vi "Network Engine.vi"(8 "error in (no error)":errorcluster, 11 "Variables":T1) -> (0 "error out":errorcluster)   [LabVIEW 2019, in "Protection and Counter Addon Engine.lvlib"]
uses:
  Protection and Counter Addon Engine.lvlib
  Types/RT Async Engine Variables.ctl
  <vilib>/NI/NIVS Inline Async API/_VS Inline Async API/Process/Process.lvclass
  <vilib>/NI/NI VeriStand Addon Network Comm/Engine/VeriStand Comm.lvclass
  Types/RT Data References.ctl
  <vilib>/NI/NIVS Inline Async API/_Data Access Engine/Data Access Engine/Types/Write.DVR.ctl
  <vilib>/NI/NIVS Inline Async API/_Data Access Engine/Access Type Classes/Write/Write.lvclass
  <vilib>/NI/NIVS Inline Async API/_Data Access Engine/Data Access Engine/Types/Read.DVR.ctl
  <vilib>/NI/NIVS Inline Async API/_Data Access Engine/Access Type Classes/Read/Read.lvclass
  Types/RT Async Engine Settings.ctl
  SubModules/Frame Protection Support/Source/Engine/Types/RT Frame Settings.ctl
  SubModules/Frame Protection Support/Source/Shared/Types/Exported Frame Type.ctl
  SubModules/Frame Protection Support/Source/Engine/Types/RT Protection Configuration.ctl
  SubModules/Frame Protection Support/Source/Shared/Types/Protection Type.ctl
  SubModules/Frame Protection Support/Source/Shared/Types/XNET Signal Configuration.ctl
  SubModules/Frame Protection Support/Source/Shared/Types/Exported Counter Settings.ctl
  SubModules/Frame Protection Support/Source/Shared/Types/Exported Event Trigger Type.ctl
  <vilib>/NI/NI VeriStand Addon Network Comm/Engine/VeriStand Comm.lvclass/VeriStand Comm.ctl
  <vilib>/NI/NIVS Inline Async API/_VS Inline Async API/Process/Process.lvclass/Process.ctl
  <vilib>/xnet/xnet.llb/XNET Frame CAN.ctl
  <vilib>/xnet/xnet.llb/XNET Frame Type CAN.ctl
  <vilib>/NI/NI VeriStand Addon Network Comm/Engine/_SubVIs/Comm Connection Engine.vi
  <vilib>/NI/NI VeriStand Addon Network Comm/Engine/_SubVIs/Comm Command Engine.vi
  <vilib>/NI/NIVS Inline Async API/_VS Inline Async API/Error Handling Process/SubVIs/Error.ConvertArray.vi
  <vilib>/NI/AMC/Read Next Message.vi
  <vilib>/NI/Tools/Keyed Array/Index.vi
  <vilib>/NI/AMC/Send Local Message.vi
  <vilib>/NI/STM/Connection Manager/TCP/Advanced/TCP Connection Manager (By Reference).vi
  <vilib>/Utility/error.llb/Clear Errors.vi
  <vilib>/NI/STM/Get Connection Reference.vi
  <vilib>/NI/STM/TCP/Get Connection Reference (TCP).vi
  <vilib>/NI/STM/Read Meta Data.vi
  <vilib>/NI/STM/TCP/Read Meta Data (TCP Ref).vi
  <vilib>/NI/Tools/Keyed Array/Add.vi
  <vilib>/NI/STM/Connection Manager/TCP/Advanced/TCP Check Connection (By Reference).vi
  <vilib>/NI/AMC/Read Termination Message.vi
  <vilib>/NI/Tools/Keyed Array/Map String.vi
  <vilib>/NI/AMC/Create Single Message.vi
  <vilib>/NI/AMC/Update Message Routing Info.vi
  <vilib>/NI/STM/SubVIs/Generate STM Error.vi
  <vilib>/NI/Tools/String/Get Case Matching.vi
  <vilib>/NI/STM/Read Message.vi
  <vilib>/NI/STM/TCP/Read Message (TCP).vi
  <vilib>/NI/AMC/Send Message.vi
  <vilib>/NI/NI VeriStand Addon Network Comm/Shared/Comm Constants.vi
  <vilib>/NI/AMC/Create Message Queue.vi
  <vilib>/NI/AMC/Globals.vi
  <vilib>/NI/STM/Write Message.vi
  <vilib>/NI/STM/TCP/Write Message (TCP).vi
  <vilib>/NI/AMC/Destroy Message Queue.vi
  <vilib>/Utility/SystemLogging/Write to System Log.vi
  <vilib>/NI/STM/TCP/Read Meta Data (TCP Clst).vi
  <vilib>/xnet/xnet.llb/XNET Write (Frame CAN).vi
  SubModules/Frame Protection Support/Source/Shared/Protection and Counter Support Shared.lvlib
  SubModules/Frame Protection Support/Source/Engine/Protection and Counter Support Engine.lvlib
  <vilib>/NI/NIVS Inline Async API/_Data Access Engine/Data Access Engine/Data Access Engine.lvclass
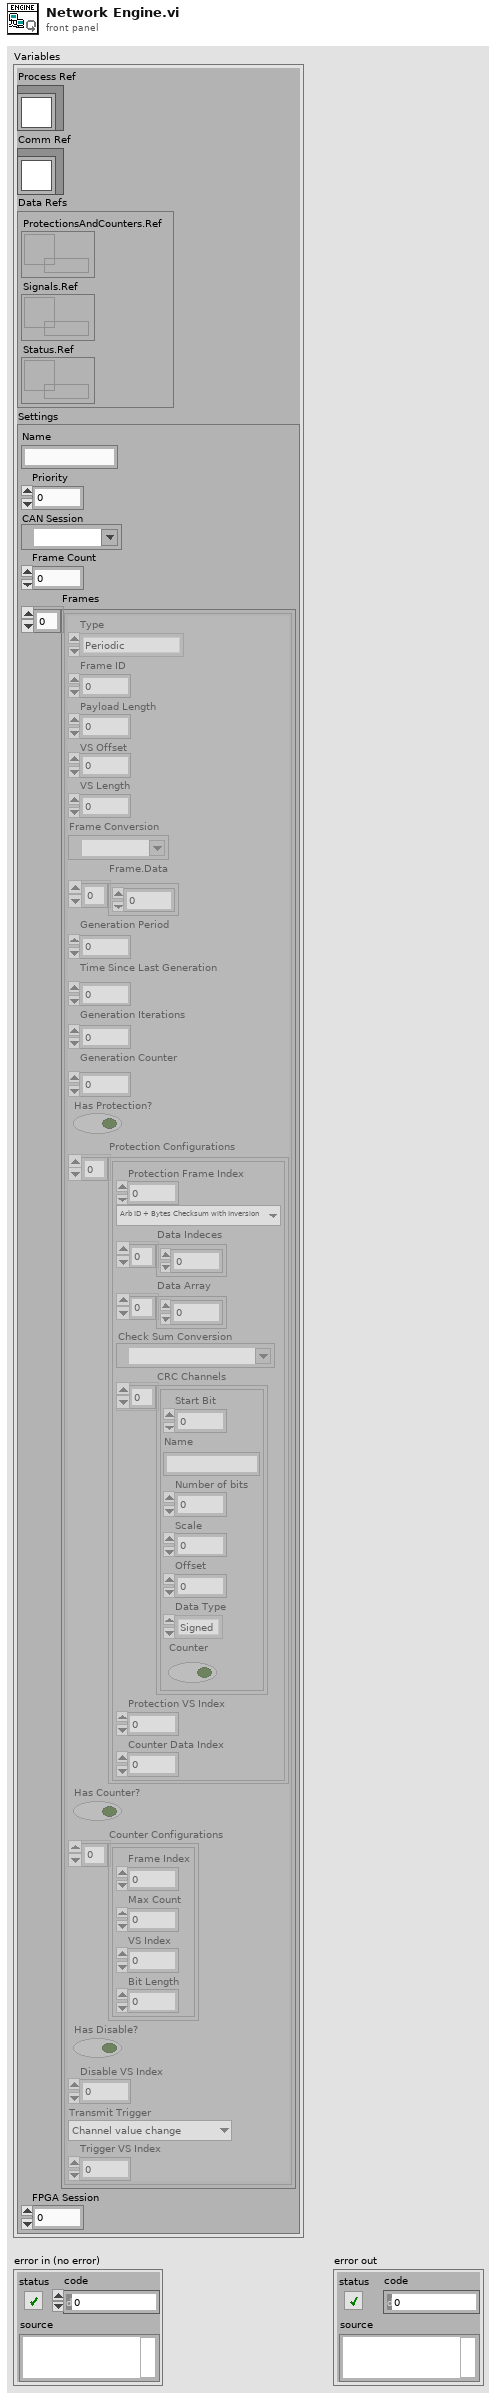
[diagram p1: front panel]
types:
  T1 = typedef "Protection and Counter Addon Engine.lvlib/RT Async Engine Variables.ctl" = cluster{"Process Ref":refnum<class "Process.lvclass">, "Comm Ref":refnum<class "VeriStand Comm.lvclass">, "Data Refs":T2, "Settings":T5}
  T2 = typedef "Protection and Counter Addon Engine.lvlib/RT Data References.ctl" = cluster{"ProtectionsAndCounters.Ref":T3, "Signals.Ref":T4, "Status.Ref":T3}
  T3 = typedef "Data Access Engine.lvlib/Data Access Engine.lvclass/Write.DVR.ctl" = refnum<data-value>
  T4 = typedef "Data Access Engine.lvlib/Data Access Engine.lvclass/Read.DVR.ctl" = refnum<data-value>
  T5 = typedef "Protection and Counter Addon Engine.lvlib/RT Async Engine Settings.ctl" = cluster{"Name":string, "Priority":i32, "CAN Session":refnum<k21>, "Frame Count":i32, "Frames":T6[], "FPGA Session":u32}
  T6 = typedef "Protection and Counter Support Engine.lvlib/RT Frame Settings.ctl" = cluster{"Type":T7, "Frame ID":u32, "Payload Length":u32, "VS Offset":i32, "VS Length":i32, "Frame Conversion":refnum<k21>, "Frame.Data":dbl[], "Generation Period":u32, "Time Since Last Generation":u32, "Generation Iterations":u32, "Generation Counter":u32, "Has Protection?":bool, "Protection Configurations":T8[], "Has Counter?":bool, "Counter Configurations":T11[], "Has Disable?":bool, "Disable VS Index":i32, "Transmit Trigger":T12, "Trigger VS Index":i32}
  T7 = typedef "Protection and Counter Support Shared.lvlib/Exported Frame Type.ctl" = enum16{"Periodic", "Event", "Periodic/Event"}
  T8 = typedef "Protection and Counter Support Engine.lvlib/RT Protection Configuration.ctl" = cluster{"Protection Frame Index":i32, "Protection Type":T9, "Data Indeces":i32[], "Data Array":dbl[], "Check Sum Conversion":refnum<k21>, "CRC Channels":T10[], "Protection VS Index":i32, "Counter Data Index":i32}
  T9 = typedef "Protection and Counter Support Shared.lvlib/Protection Type.ctl" = enum16{"Arb ID + Bytes Checksum with Inversion", "Arb ID + Bytes CRC with Inversion", "Reversed Raw Signal Checksum with Inversion", "Concatenated Two's Compliment"}
  T10 = typedef "Protection and Counter Support Shared.lvlib/XNET Signal Configuration.ctl" = cluster{"Start Bit":i32, "Name":string, "Number of bits":i32, "Scale":dbl, "Offset":dbl, "Data Type":u32, "Counter":bool}
  T11 = typedef "Protection and Counter Support Shared.lvlib/Exported Counter Settings.ctl" = cluster{"Frame Index":i32, "Max Count":dbl, "VS Index":i32, "Bit Length":i64}
  T12 = typedef "Protection and Counter Support Shared.lvlib/Exported Event Trigger Type.ctl" = enum16{"Channel value change", "Trigger channel (not zero)", "Channel value change or trigger channel (not zero)", "Trigger channel (any value change)", "Channel value change or trigger channel (any value change)"}
  T13 = typedef "XNET Frame CAN.ctl" = cluster{"timestamp":timestamp, "payload":u8[], "identifier":u32, "type":T14, "extended?":bool, "echo?":bool}
  T14 = typedef "XNET Frame Type CAN.ctl" = u8
  T15 = typedef "NI VeriStand Addon Network Comm.lvlib/VeriStand Comm.lvclass/Response Information.ctl" = cluster{"response name":string, "responseQ":string}
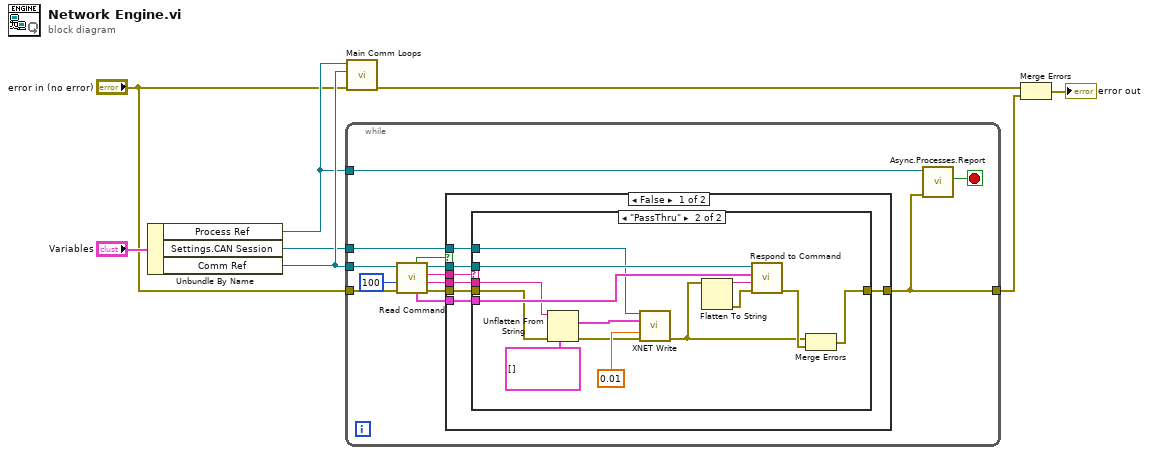
[diagram p0: block diagram]
diagram:
  n1 = Unbundle By Name("Variables") -> ("Process Ref"=w3:refnum<class "Process.lvclass">, "Settings.CAN Session"=w4:refnum<k21>, "Comm Ref"=w5:refnum<class "VeriStand Comm.lvclass">)
  n2 = while {
    tunnel: w3 -> [w21]
    tunnel: "error in (no error)" -> [w19]
    tunnel: w5 -> [w18]
    tunnel: w4 -> [w15]
    tunnel: [w12] -> w6
    stop <- w20 stop-if-true
    n3 = call <vilib>:"Read Command.vi"("error in (no error)"=w19, "timeout (100 ms)"=100, "VeriStand Comm in"=w18) -> ("error out"=w13:errorcluster, "message value"=w14:string, "message name"=w11:string, "VeriStand Comm out"=w17:refnum<class "VeriStand Comm.lvclass">, "ResponseInfo"=w16:T15, "timed out?"=w10:bool)  [unwired: 3 in]
    n4 = case shown="False" w10 {
      tunnel: w17 -> [w28 _]
      tunnel: w16 -> [w27 _]
      tunnel: w15 -> [w26 _]
      tunnel: w14 -> [w25 _]
      tunnel: w13 -> [w24 w44]
      tunnel: [w23 w44] -> w12
      tunnel: w11 -> [w22 _]
      frame False {
        n5 = case shown="\"PassThru\"" w22 {
          tunnel: w28 -> [_ w43]
          tunnel: w27 -> [_ w42]
          tunnel: w26 -> [_ w40]
          tunnel: w25 -> [_ w39]
          tunnel: w24 -> [w29 w38]
          tunnel: [w29 w33] -> w23
          frame "", Default {
          }
          frame "PassThru" {
            n6 = Unflatten From String(type=T13[] [] ("data"), binary string=w39, error in (no error)=w38) -> (value=w35:T13[], error out=w37:errorcluster)  [unwired: 2 in, 1 out]
            n7 = call-poly <vilib>:"XNET Write.vi"("session in"=w40, "data"=w35, "timeout (10)"=0.01, "error in (no error)"=w37) -> ("error out"=w31:errorcluster)  [unwired: 10 in, 1 out]
            n8 = Flatten To String(anything=w31) -> (data string=w32:string, error out=w30:errorcluster)  [unwired: 3 in, 1 out]
            n9 = call <vilib>:"Respond to Command.vi"("error in (no error)"=w30, "message value"=w32, "ResponseInfo"=w42, "VeriStand Comm in"=w43) -> ("error out"=w34:errorcluster)  [unwired: 5 in, 2 out]
            n10 = Merge Errors(w31, w34) -> (w33:errorcluster)
          }
        }
      }
      frame True {
      }
    }
    n11 = call <vilib>:"Async.Processes.Report.vi"("Error"=w12, "Process in"=w21) -> ("Stop"=w20:bool)  [unwired: 8 in, 1 out]
  }
  n12 = call <vilib>:"Main Comm Loops.vi"("error in (no error)"="error in (no error)", "Comm.lvclass"=w5, "Process"=w3) -> ("error out"=w7:errorcluster)  [unwired: 8 in]
  n13 = Merge Errors(w7, w6) -> (→"error out":errorcluster)
